vi "fit -- freq vs T controller.vi"(0 "time points":dbl[](array[numeric]), 1 "varshni win (relative)":dbl=1.25, 2 "fit using":T1=enum."varshni", 5 "temperature points":dbl[](array[numeric]), 9 "frequency points":dbl[](array[numeric]), 11 "cursor bracket: Time":T2={"left"=2378.60310421286, "right "=2421.6740576496672, "center"=2421.6740576496672, "window"=2421.6740576496672, "cursors"=[], "relative"=0, "absolute"=0, "fixed vertical offset"=2421.6740576496672, "vertical offset"=2421.6740576496672, "skew"=2421.6740576496672, "default window frac"=2421.6740576496672, "kind"=enum."skewed", "skew.left"=2421.6740576496672, "skew.right"=2421.6740576496672, "Plot ref"=refnum, "wing order"=enum."back"}) -> (3 "best fit parameters":dbl[](array[numeric])=[1510.033618014085, -0.06734487332989668, -59.94387240978006], 4 "fit function name":string="fit function - varshni3.vi", 13 "fit points before":i32=434, 14 "fit points after":i32=434)   [LabVIEW 2021]
uses:
  cursor winow.ctl
  fit function selector control.ctl
  <vilib>/Analysis/6fits.llb/Curve Fitting Criteria.ctl
  Q -- check range.vi
  Q - not nan and not zero.vi
  <vilib>/gmath/NumericalOptimization/Nonlinear Curve Fit LM.vi
  <vilib>/Analysis/NI_AALPro.lvlib
  <vilib>/gmath/NI_Gmath.lvlib
  <vilib>/Analysis/NI_AALBase.lvlib
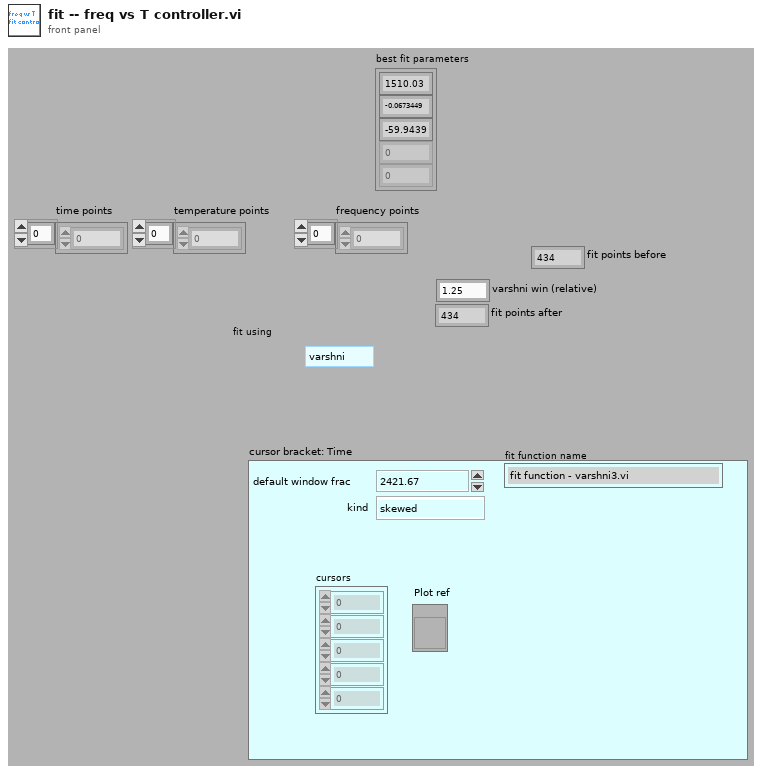
[diagram p1: front panel]
types:
  T1 = typedef "fit function selector control.ctl" = enum16{"linear", "varshni", "varshni5", "LogMinusT", "hyperbola", "einstein", "sine", "sine2theta", "cos2theta"}
  T2 = typedef "cursor winow.ctl" = cluster{"left":dbl, "right ":dbl, "center":dbl, "window":dbl, "cursors":i32[], "relative":i32, "absolute":i32, "fixed vertical offset":dbl, "vertical offset":dbl, "skew":dbl, "default window frac":dbl, "kind":enum16{"symmetric", "skewed", "fancy"}, "skew.left":dbl, "skew.right":dbl, "Plot ref":refnum<vi>, "wing order":enum16{"forw", "back"}}
  T3 = typedef "NI_AALPro.lvlib/Curve Fitting Criteria.ctl" = u16
  T4 = cluster{"model":string, "Parameters":string[], "x":string}
  T5 = typedef "NI_Gmath.lvlib/LM model function reference.ctl" = refnum<vi>
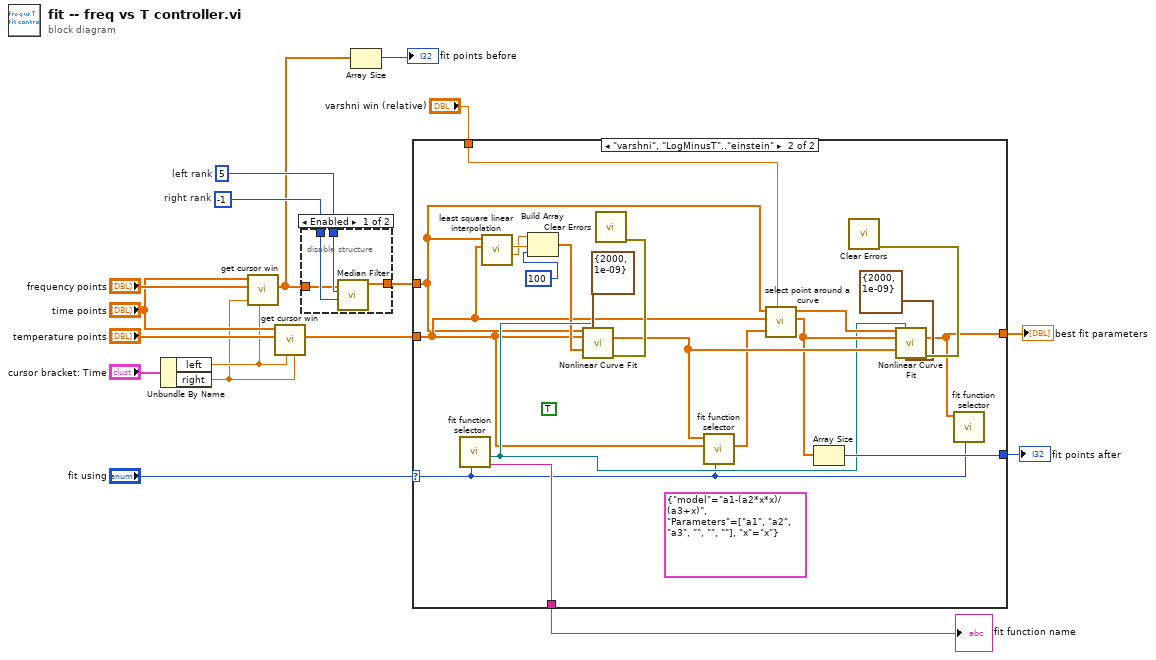
[diagram p0: block diagram]
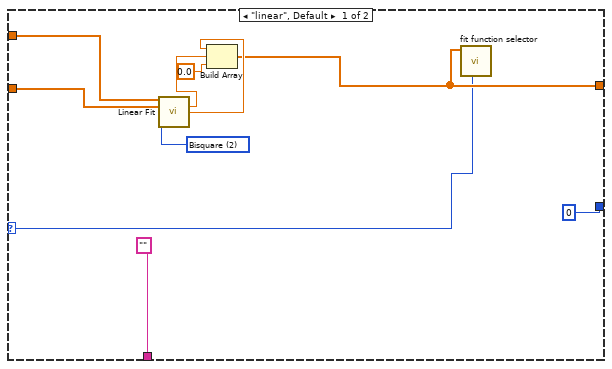
[diagram p3: hidden frame]
diagram:
  w10 = -1  # right rank
  w11 = 5  # left rank
  n1 = Unbundle By Name("cursor bracket: Time") -> ("left"=w7:dbl, "right"=w6:dbl)
  n2 = call "get cursor win.vi"("right"=w6, "left"=w7, "freq"="frequency points", "time points"="time points") -> ("freq out"=w8:dbl[])  [unwired: 7 in]
  n3 = call "get cursor win.vi"("right"=w6, "left"=w7, "freq"="temperature points", "time points"="time points") -> ("freq out"=w2:dbl[])  [unwired: 7 in]
  n4 = disable-structure shown="Enabled" {
    disable-tunnel: w11 -> [w21 _]
    disable-tunnel: w10 -> [w20 _]
    disable-tunnel: w8 -> [w19 w22]
    disable-tunnel: [w18 w22] -> w1
    frame Enabled {
      n5 = call <vilib>:"Median Filter.vi"("right rank"=w20, "left rank"=w21, "X"=w19) -> ("Filtered X"=w18:dbl[])  [unwired: 7 in, 1 out]
    }
    frame Disabled {
    }
  }
  n6 = Array Size(array=w8) -> (size(s)=→"fit points before":i32)
  n7 = case shown="\"varshni\", \"LogMinusT\"..\"einstein\"" "fit using" {
    selector: "fit using" -> [w23 w33]
    tunnel: w1 -> [w30 w35]
    tunnel: w2 -> [w31 w36]
    tunnel: [w26 w43] -> w5
    tunnel: "varshni win (relative)" -> [_ w44]
    tunnel: [0 w42] -> w4
    tunnel: ["" w41] -> w3
    frame "linear", Default {
      w32 = T3 2 items=["Least Square", "Least Absolute Residual", "Bisquare"] ("method")
      n8 = call <vilib>:"Linear Fit.vi"("Y"=w30, "X"=w31, "method"=w32) -> ("slope"=w29:dbl, "intercept"=w27:dbl)  [unwired: 8 in, 3 out]
      n9 = Build Array(w27, w29, 0.0) -> (w26:dbl[])
      n10 = call "fit function selector.vi"("fit using"=w23, "best fit parameters"=w26) -> ()  [unwired: 7 in, 3 out]
    }
    frame "varshni", "LogMinusT".."einstein" {
      (unwired) T4 {"model"="a1-(a2*x*x)/(a3+x)", "Parameters"=["a1", "a2", "a3", "", "", ""], "x"="x"} ("model description")
      (unwired) TRUE
      n11 = call "fit function selector.vi"("fit using"=w33) -> ("fit function name"=w41:string, "vi reference"=w40:T5)  [unwired: 8 in, 1 out]
      n12 = call "least square linear interpolation.vi"("X"=w36, "Y"=w35) -> ("intercept"=w34:dbl, "slope"=w37:dbl)  [unwired: 6 in, 2 out]
      n13 = Build Array(w34, w37, 100) -> (w38:dbl[])
      n14 = call-poly <vilib>:"Nonlinear Curve Fit.vi"("Y"=w35, "f(x,a)"=w40, "X"=w36, "initial parameters"=w38, "termination"=cluster{"max iteration":i32, "tolerance":dbl} {"max iteration"=2000, "tolerance"=1e-09}) -> ("best fit parameters"=w47:dbl[], "error out"=w51:errorcluster)  [unwired: 5 in, 4 out]
      n15 = call <vilib>:"Clear Errors.vi"("error in (no error)"=w51) -> ()  [unwired: 5 in, 2 out]
      n16 = call "fit function selector.vi"("fit using"=w33, "temperature"=w36, "best fit parameters"=w47) -> ("freq out"=w39:dbl[])  [unwired: 6 in, 2 out]
      n17 = call "select point around a curve.vi"("freq  ref curve"=w39, "window"=w44, "temperature"=w36, "freq"=w35) -> ("temperature  out"=w46:dbl[], "freq out"=w45:dbl[])  [unwired: 6 in]
      n18 = Array Size(array=w46) -> (size(s)=w42:i32)
      n19 = call-poly <vilib>:"Nonlinear Curve Fit.vi"("Y"=w45, "f(x,a)"=w40, "X"=w46, "initial parameters"=w47, "termination"=cluster{"max iteration":i32, "tolerance":dbl} {"max iteration"=2000, "tolerance"=1e-09}) -> ("best fit parameters"=w43:dbl[], "error out"=w49:errorcluster)  [unwired: 5 in, 4 out]
      n20 = call <vilib>:"Clear Errors.vi"("error in (no error)"=w49) -> ()  [unwired: 5 in, 2 out]
      n21 = call "fit function selector.vi"("fit using"=w33, "best fit parameters"=w43) -> ()  [unwired: 7 in, 3 out]
    }
  }
  "best fit parameters" <- w5
  "fit points after" <- w4
  "fit function name" <- w3
